vi "Set Plot Names.vi"(8 "错误输入":cluster{"状态":bool, "代码":i32, "源":string}, 10 "曲线名":string[](array[string]), 11 "图形引用":refnum<vi>) -> (0 "错误输出":cluster{"状态":bool, "代码":i32, "源":string})   [LabVIEW 2012]
doc: "该VI用于在波形图表或波形图上设置曲线名。"
uses:
  <vilib>/Utility/error.llb/Error Cluster From Error Code.vi
  <vilib>/ErrorRing/Error Ring.xnode
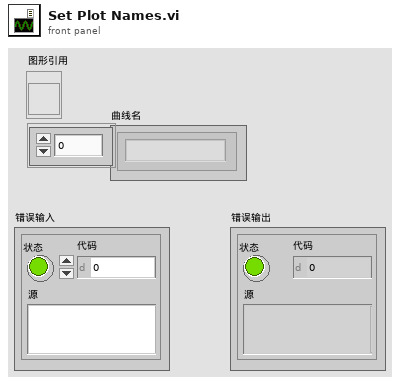
[diagram p1: front panel]
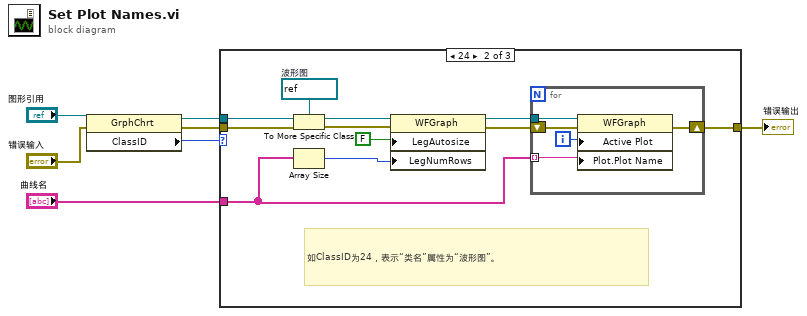
[diagram p0: block diagram]
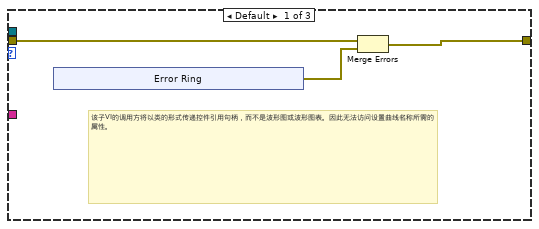
[diagram p2: hidden frame]
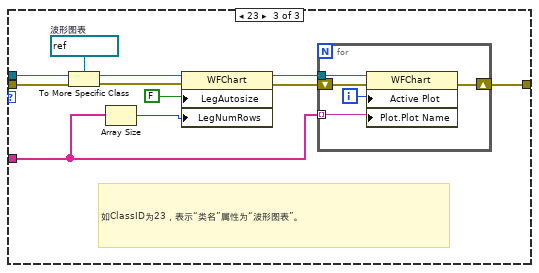
[diagram p3: hidden frame]
diagram:
  n1 = property on="属性节点" class="GrphChrt"(reference="图形引用", error in="错误输入") -> (reference out=w5:refnum<vi>, error out=w6:errorcluster, "ClassID"=w1:u32)
  n2 = case shown="24" w1 {
    tunnel: w6 -> [w10 w19 w35]
    tunnel: w5 -> [_ w20 w36]
    tunnel: "曲线名" -> [_ w15 w31]
    tunnel: [w9 w17 w33] -> w3
    frame Default {
      # "该子VI的调用方将以类的形式传递控件引用句柄，而不是波形图或波形图表。因此无法访问设置曲线名称所需的属性。"
      n3 = xnode "Error Ring"() -> ("错误输出"=w8:errorcluster)
      n4 = Merge Errors ("合并错误")(w10, w8) -> (w9:errorcluster)
    }
    frame 24 {
      w25 = refnum<vi> refnum  # 波形图
      # "如ClassID为24，表示“类名”属性为“波形图”。"
      n5 = To More Specific Class ("转换为特定的类")(target class=w25, reference=w20, error in=w19) -> (specific class reference=w23:refnum<vi>, error out=w24:errorcluster)
      n6 = Array Size ("数组大小")(array=w15) -> (size(s)=w16:i32)
      n7 = property on="属性节点" class="WFGraph"(reference=w23, error in=w24, "LegAutosize"=FALSE ("图例:自动调整大小"), "LegNumRows"=w16) -> (reference out=w21:refnum<vi>, error out=w18:errorcluster)
      n8 = for {
        tunnel: w21 -> [w30]
        shift-right: [w28] -> w17
        shift-left: w18 -> [w29]
        tunnel: w15 -> [w26] mode=indexing
        i -> [w27]
        n9 = property on="属性节点" class="WFGraph"(reference=w30, error in=w29, "Active Plot"=w27, "Plot.Plot Name"=w26) -> (error out=w28:errorcluster)  [unwired: 1 out]
      }
    }
    frame 23 {
      w41 = refnum<vi> refnum  # 波形图表
      # "如ClassID为23，表示“类名”属性为“波形图表”。"
      n10 = To More Specific Class ("转换为特定的类")(target class=w41, reference=w36, error in=w35) -> (specific class reference=w39:refnum<vi>, error out=w40:errorcluster)
      n11 = Array Size ("数组大小")(array=w31) -> (size(s)=w32:i32)
      n12 = property on="属性节点" class="WFChart"(reference=w39, error in=w40, "LegAutosize"=FALSE ("图例:自动调整大小"), "LegNumRows"=w32) -> (reference out=w37:refnum<vi>, error out=w34:errorcluster)
      n13 = for {
        tunnel: w37 -> [w46]
        shift-right: [w44] -> w33
        shift-left: w34 -> [w45]
        tunnel: w31 -> [w42] mode=indexing
        i -> [w43]
        n14 = property on="属性节点" class="WFChart"(reference=w46, error in=w45, "Active Plot"=w43, "Plot.Plot Name"=w42) -> (error out=w44:errorcluster)  [unwired: 1 out]
      }
    }
  }
  "错误输出" <- w3
